vi "P2_1_Fibonacci.vi"() -> ()   [LabVIEW 2020]
panel:
  out "Serie de Fibonacci":dbl[](array[numeric])
  out "Indicador escalar":i32
  in  "No. de elementos":i32
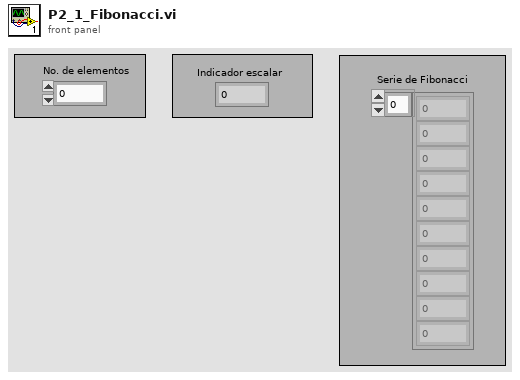
[diagram p1: front panel]
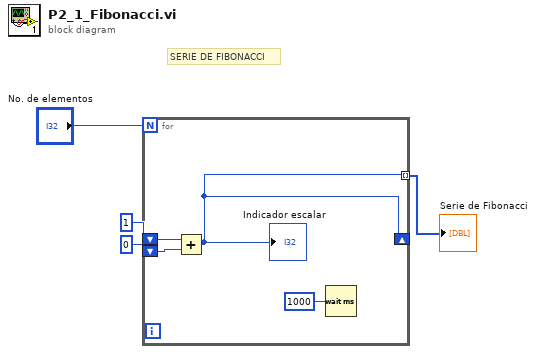
[diagram p0: block diagram]
diagram:
  # "SERIE DE FIBONACCI"
  n1 = for {
    N: "No. de elementos" -> [_]
    shift-right: [w5] -> _
    shift-left: 1 -> [w7]
    shift-left: 0 -> [w6]
    tunnel: [w5] -> w1 mode=indexing
    n2 = Add(x=w7, y=w6) -> (x+y=w5:i32)
    "Indicador escalar" <- w5
    n3 = Wait (ms)(milliseconds to wait=u32 1000) -> ()  [unwired: 1 out]
  }
  "Serie de Fibonacci" <- w1
